vi "CH1_Save_Header_Python.vi"() -> ()   [LabVIEW 2018]
uses:
  RxTx/RxTx.lvclass
  Save Image/Save Image.lvclass
  Channel/Channel.lvclass
panel:
  out "error out":errorcluster
  in  "Save Image out":refnum<class "Save Image.lvclass">
  in  "RxTx.lvclass":refnum<class "RxTx.lvclass">
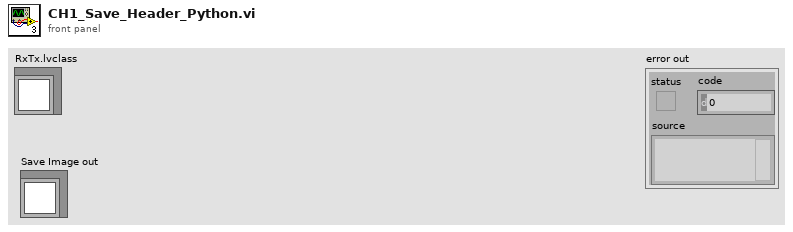
[diagram p1: front panel]
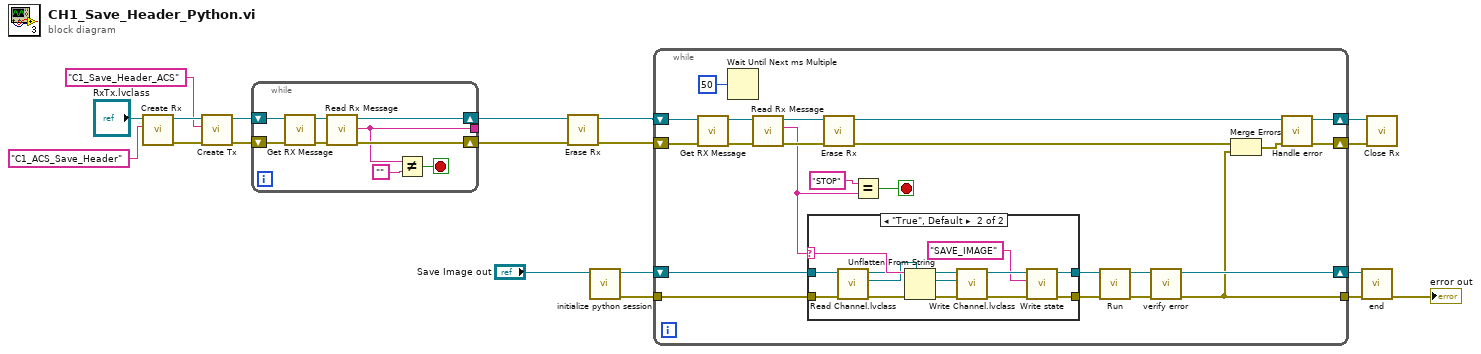
[diagram p0: block diagram]
diagram:
  n1 = call "Create Rx.vi"("Reader Name"="C1_ACS_Save_Header", "RxTx in"="RxTx.lvclass") -> ("error out"=w6:errorcluster, "RxTx out"=w9:refnum<class "RxTx.lvclass">)  [unwired: 8 in]
  n2 = call "Create Tx.vi"("error in (no error)"=w6, "Writer Name"="C1_Save_Header_ACS" ("Reader Name"), "RxTx in"=w9) -> ("error out"=w7:errorcluster, "RxTx out"=w8:refnum<class "RxTx.lvclass">)  [unwired: 7 in]
  n3 = while {
    shift-right: [w26] -> w14
    shift-left: w7 -> [w28]
    shift-right: [w25] -> w11
    shift-left: w8 -> [w23]
    tunnel: [w20] -> _
    stop <- w21 stop-if-true
    n4 = call "Get RX Message.vi"("error in (no error)"=w28, "RxTx in"=w23) -> ("error out"=w27:errorcluster, "RxTx out"=w24:refnum<class "RxTx.lvclass">)  [unwired: 7 in, 1 out]
    n5 = call "Read Rx Message.vi"("error in (no error)"=w27, "RxTx in"=w24) -> ("error out"=w26:errorcluster, "Rx Message"=w20:string, "RxTx out"=w25:refnum<class "RxTx.lvclass">)  [unwired: 7 in]
    n6 = Not Equal?(x=w20, y="") -> (x != y?=w21:bool)
  }
  n7 = call "Erase Rx.vi"("error in (no error)"=w14, "RxTx in"=w11) -> ("error out"=w13:errorcluster, "RxTx out"=w12:refnum<class "RxTx.lvclass">)  [unwired: 8 in]
  n8 = call "initialize python session.vi"("Save Image in"="Save Image out") -> ("error out"=w3:errorcluster, "Save Image out"=w17:refnum<class "Save Image.lvclass">)  [unwired: 9 in]
  n9 = while {
    shift-right: [w37] -> w4
    shift-left: w12 -> [w51]
    shift-right: [w30] -> w15
    shift-left: w17 -> [w44]
    shift-right: [w36] -> w1
    shift-left: w13 -> [w50]
    tunnel: w3 -> [w38]
    tunnel: [w29] -> w2
    stop <- w39 stop-if-true
    n10 = call "Get RX Message.vi"("error in (no error)"=w50, "RxTx in"=w51) -> ("error out"=w48:errorcluster, "RxTx out"=w49:refnum<class "RxTx.lvclass">)  [unwired: 7 in, 1 out]
    n11 = Wait Until Next ms Multiple(millisecond multiple=u32 50) -> ()  [unwired: 1 out]
    n12 = call "Read Rx Message.vi"("error in (no error)"=w48, "RxTx in"=w49) -> ("error out"=w42:errorcluster, "Rx Message"=w40:string, "RxTx out"=w43:refnum<class "RxTx.lvclass">)  [unwired: 7 in]
    n13 = case shown="\"True\", Default" w40 {
      selector: w40 -> [_ w66]
      tunnel: [w53 w57] -> w46
      tunnel: [w52 w55] -> w45
      tunnel: w38 -> [w52 w64]
      tunnel: w44 -> [w53 w65]
      frame "", "STOP" {
      }
      frame "True", Default {
        n14 = call-dynamic "Read Channel.lvclass.vi"("error in (no error)"=w64, "Save Image in"=w65) -> ("error out"=w63:errorcluster, "Channel.lvclass"=w60:refnum<class "Channel.lvclass">, "Save Image out"=w61:refnum<class "Save Image.lvclass">)  [unwired: 7 in]
        n15 = Unflatten From String(type=w60, binary string=w66, error in (no error)=w63) -> (value=w59:refnum<class "Channel.lvclass">, error out=w62:errorcluster)  [unwired: 2 in, 1 out]
        n16 = call-dynamic "Write Channel.lvclass.vi"("error in (no error)"=w62, "Channel.lvclass"=w59, "Save Image in"=w61) -> ("error out"=w56:errorcluster, "Save Image out"=w58:refnum<class "Save Image.lvclass">)  [unwired: 7 in]
        n17 = call "Write state.vi"("error in (no error)"=w56, "String"="SAVE_IMAGE" ("Reader Name"), "Save Image in"=w58) -> ("error out"=w55:errorcluster, "Save Image out"=w57:refnum<class "Save Image.lvclass">)  [unwired: 7 in]
      }
    }
    n18 = call "Erase Rx.vi"("error in (no error)"=w42, "RxTx in"=w43) -> ("error out"=w33:errorcluster, "RxTx out"=w35:refnum<class "RxTx.lvclass">)  [unwired: 8 in]
    n19 = Equal?(x="STOP" ("Reader Name"), y=w40) -> (x = y?=w39:bool)
    n20 = call "Run.vi"("error in (no error)"=w45, "Save Image in"=w46) -> ("error out"=w32:errorcluster, "Save Image out"=w31:refnum<class "Save Image.lvclass">)  [unwired: 8 in]
    n21 = call "verify error.vi"("error in (no error)"=w32, "Save Image in"=w31) -> ("error out"=w29:errorcluster, "Save Image out"=w30:refnum<class "Save Image.lvclass">)  [unwired: 8 in]
    n22 = Merge Errors(w33, w29) -> (w34:errorcluster)
    n23 = call "Handle error.vi"("error in (no error)"=w34, "RxTx in"=w35) -> ("error out"=w36:errorcluster, "RxTx out"=w37:refnum<class "RxTx.lvclass">)  [unwired: 8 in]
  }
  n24 = call "end.vi"("error in (no error)"=w2, "Save Image in"=w15) -> ("error out"=→"error out":errorcluster)  [unwired: 8 in, 1 out]
  n25 = call "Close Rx.vi"("error in (no error)"=w1, "RxTx in"=w4) -> ()  [unwired: 8 in, 2 out]
